vi "Get Valid Event Time.vi"(1 "Event Time In":timestamp) -> (0 "Event Time Out":timestamp)   [LabVIEW 2020, in "Composed Log.lvlib" / "LoggerReference.lvclass"]
uses:
  <vilib>/gpm_packages/@cs/event-logger/Source/Composed Log/LoggerReference/LoggerReference.lvclass
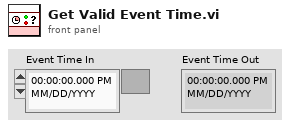
[diagram p1: front panel]
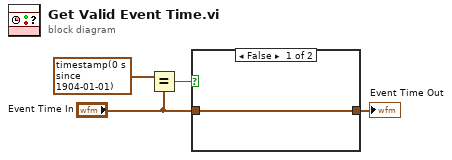
[diagram p0: block diagram]
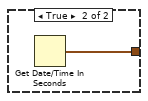
[diagram p2: hidden frame]
diagram:
  n1 = Equal?(x=timestamp(0 s since 1904-01-01), y="Event Time In") -> (x = y?=w3:bool)
  n2 = case shown="False" w3 {
    tunnel: "Event Time In" -> [w5 _]
    tunnel: [w5 w6] -> w1
    frame False {
    }
    frame True {
      n3 = Get Date/Time In Seconds() -> (seconds since 1Jan1904=w6:timestamp)
    }
  }
  "Event Time Out" <- w1
